vi "process camera timestamp.vi"(0 "Progress:":refnum<vi>, 1 "Use Harp converted .csv file\nto timestamp the file:":bool, 2 "abort":refnum<vi>, 3 "Register Address:":refnum<vi>, 4 "cam .csv":path, 5 "CameraBitPosition":refnum<vi>, 6 "don't ask":bool, 7 "harp .bin":path) -> (8 "error":string="Frames on Harp file: ")   [LabVIEW 2010]
panel:
  out "Frames Acquired":i32
  out "Numeric":i32
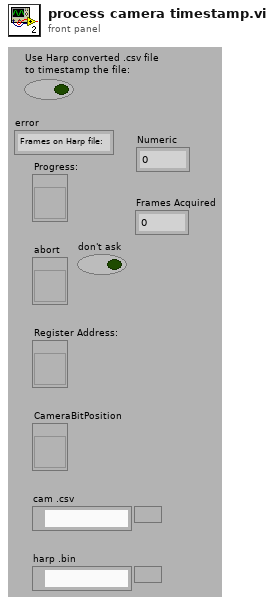
[diagram p1: front panel]
types:
  T1 = enum8{"Enabled", "Disabled", "Disabled and Grayed Out"}
  T2 = enum16{"open", "replace", "create", "open or create", "replace or create", "replace or create with confirmation"}
  T3 = enum16{"Left Button", "Center Button", "Right Button", "Window Close"}
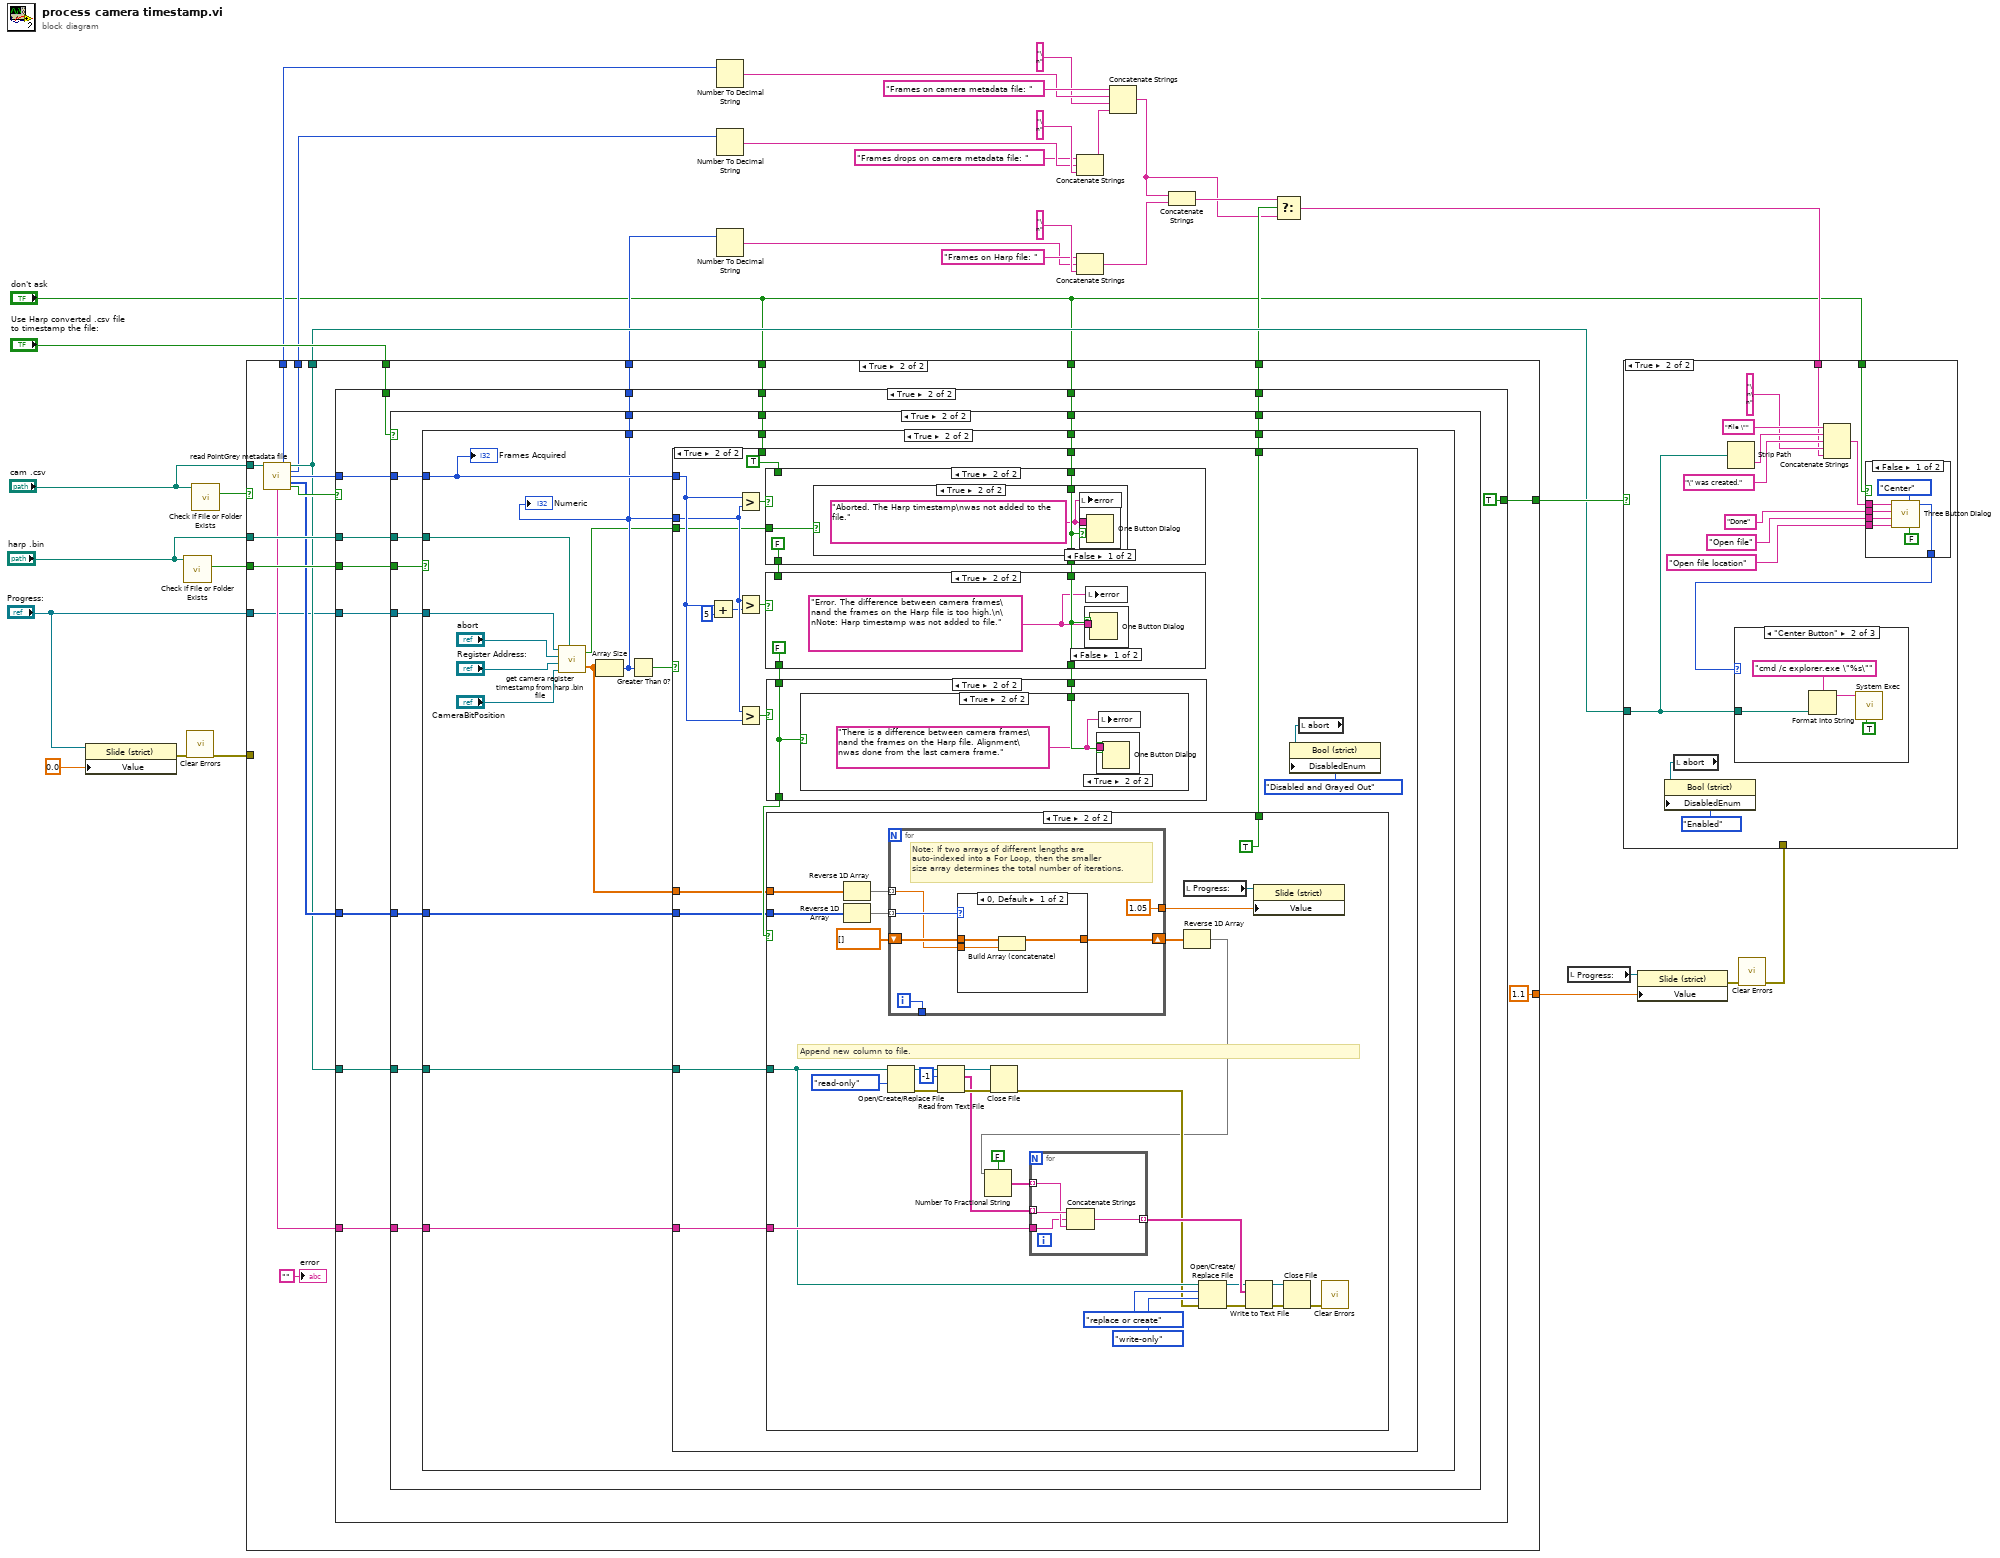
[diagram p0: block diagram]
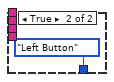
[diagram p3: hidden frame]
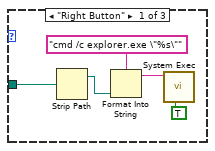
[diagram p4: hidden frame]
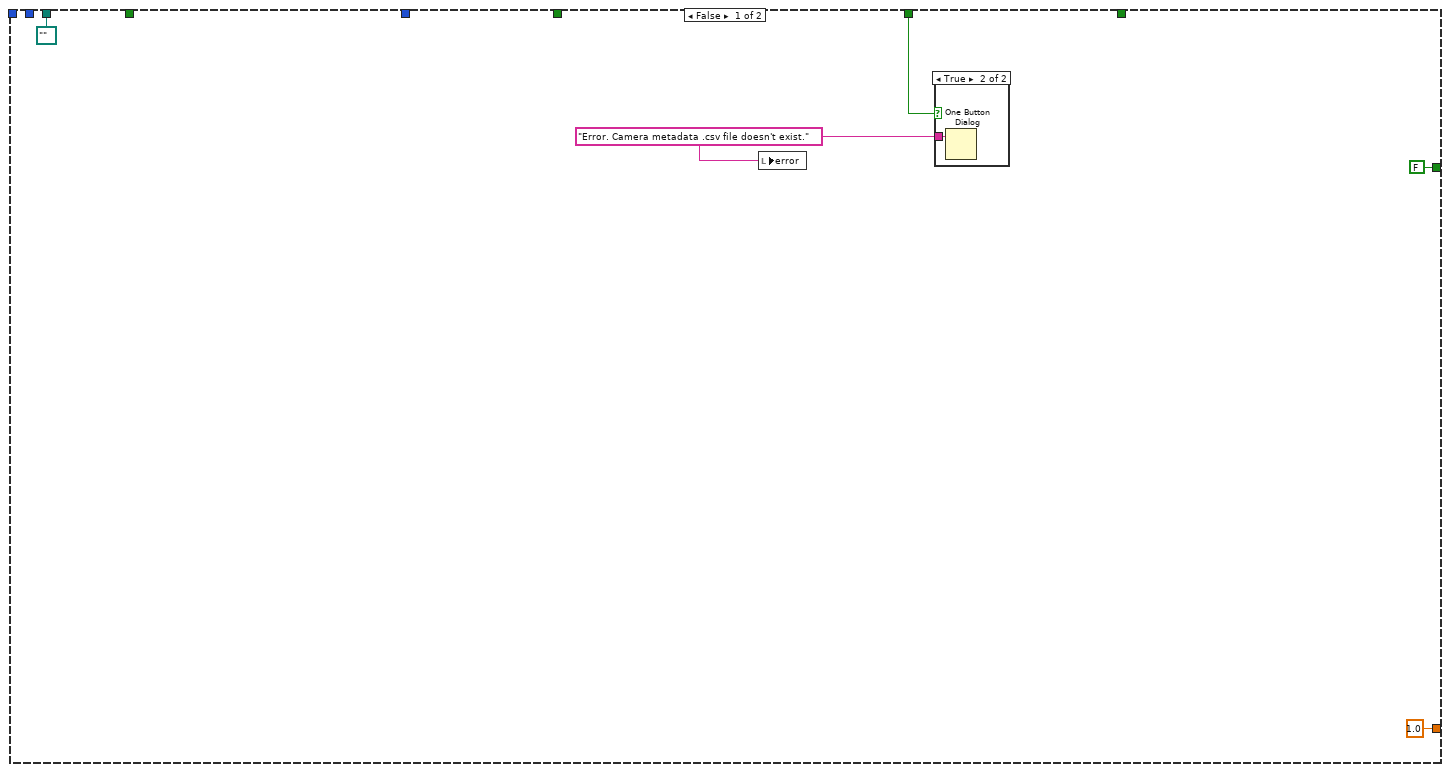
[diagram p6: hidden frame]
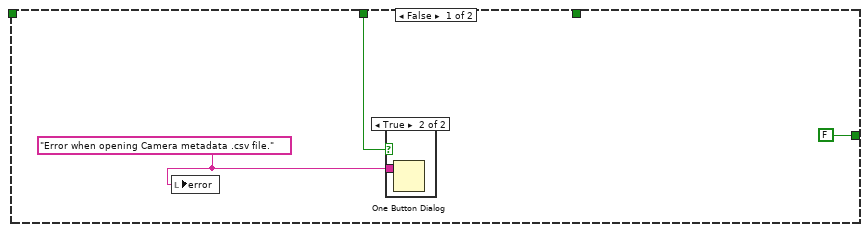
[diagram p8: hidden frame]
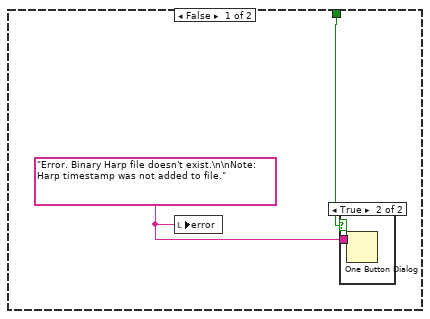
[diagram p11: hidden frame]
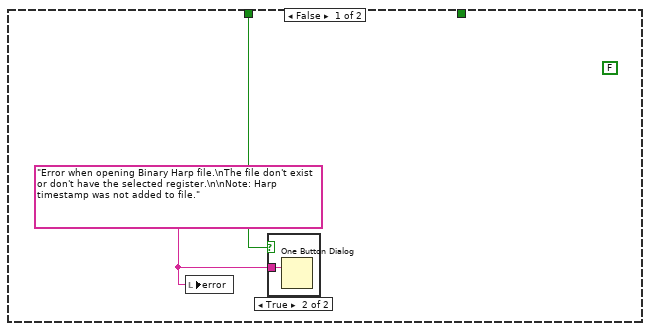
[diagram p13: hidden frame]
diagram:
  n1 = property class="Slide (strict)"(reference="Progress:", "Value"=0.0) -> (error out=w27:errorcluster)  [unwired: 1 in, 1 out]
  n2 = call <vilib>:"Check if File or Folder Exists.vi"("path"="harp .bin") -> ("file or folder exists?"=w30:bool)  [unwired: 8 in, 2 out]
  n3 = call <vilib>:"Clear Errors.vi"("error in (no error)"=w27) -> ("error out"=w26:errorcluster)  [unwired: 6 in]
  n4 = call <vilib>:"Check if File or Folder Exists.vi"("path"="cam .csv") -> ("file or folder exists?"=w33:bool)  [unwired: 8 in, 2 out]
  n5 = case shown="True" w33 {
    tunnel: "harp .bin" -> [_ w53]
    tunnel: "cam .csv" -> [_ w59]
    tunnel: "Use Harp converted .csv file\nto timestamp the file:" -> [_ w57]
    tunnel: [FALSE w56] -> w29
    tunnel: w30 -> [_ w55]
    tunnel: [path "" ("Created Csv File") w50] -> w28
    tunnel: w26 -> [_ _]
    tunnel: "Progress:" -> [_ w49]
    tunnel: [_ w48] -> w23
    tunnel: [_ w47] -> w16
    tunnel: [1.0 ("Value") 1.1 ("Value")] -> w10
    tunnel: [_ w45] -> w4
    tunnel: [_ w44] -> w2
    tunnel: "don't ask" -> [_ w43]
    tunnel: "don't ask" -> [w35 w42]
    frame False {
      w36 = "Error. Camera metadata .csv file doesn't exist." ("message")
      n6 = local write "error"(w36) -> ()
      n7 = case shown="True" w35 {
        tunnel: w36 -> [_ w40]
        frame False {
        }
        frame True {
          n8 = One Button Dialog(message=w40) -> ()  [unwired: 1 in, 1 out]
        }
      }
    }
    frame True {
      n9 = call "read PointGrey metadata file.vi"("PointGrey metadata file path"=w59) -> ("Frames On File"=w44:i32, "Created Csv File"=w50:path, "Frame Drops"=w45:i64, "Frames Acquired"=w54:i32, "FrameCounter (processed)"=w52:i64[], "Separation Character"=w51:string, "File Has Data"=w58:bool)  [unwired: 8 in]
      n10 = case shown="True" w58 {
        tunnel: w57 -> [_ w76]
        tunnel: [FALSE TRUE] -> w56
        tunnel: w55 -> [_ w75]
        tunnel: w54 -> [_ w66]
        tunnel: w53 -> [_ w74]
        tunnel: w52 -> [_ w73]
        tunnel: w50 -> [_ w72]
        tunnel: w51 -> [_ w71]
        tunnel: w49 -> [_ w69]
        tunnel: [_ w68] -> w48
        tunnel: [_ w67] -> w47
        tunnel: w43 -> [_ w65]
        tunnel: w42 -> [w60 w64]
        frame False {
          w61 = "Error when opening Camera metadata .csv file." ("message")
          n11 = local write "error"(w61) -> ()
          n12 = case shown="True" w60 {
            tunnel: w61 -> [_ w63]
            frame False {
            }
            frame True {
              n13 = One Button Dialog(message=w63) -> ()  [unwired: 1 in, 1 out]
            }
          }
        }
        frame True {
          n14 = case shown="True" w76 {
            tunnel: w75 -> [_ w87]
            tunnel: w66 -> [_ w86]
            tunnel: w74 -> [_ w85]
            tunnel: w73 -> [_ w84]
            tunnel: w72 -> [_ w83]
            tunnel: w71 -> [_ w82]
            tunnel: w69 -> [_ w81]
            tunnel: [_ w80] -> w68
            tunnel: [_ w79] -> w67
            tunnel: w65 -> [_ w78]
            tunnel: w64 -> [_ w77]
            frame False {
            }
            frame True {
              n15 = case shown="True" w87 {
                tunnel: w86 -> [_ w97]
                tunnel: w85 -> [_ w102]
                tunnel: w84 -> [_ w93]
                tunnel: w83 -> [_ w100]
                tunnel: w82 -> [_ w99]
                tunnel: w81 -> [_ w98]
                tunnel: [_ w96] -> w80
                tunnel: [_ w95] -> w79
                tunnel: w78 -> [_ w92]
                tunnel: w77 -> [w88 w91]
                frame False {
                  w89 = "Error. Binary Harp file doesn't exist.\n\nNote: Harp timestamp was not added to file." ("message")
                  n16 = local write "error"(w89) -> ()
                  n17 = case shown="True" w88 {
                    tunnel: w89 -> [_ w90]
                    frame False {
                    }
                    frame True {
                      n18 = One Button Dialog(message=w90) -> ()  [unwired: 1 in, 1 out]
                    }
                  }
                }
                frame True {
                  n19 = call "get camera register timestamp from harp .bin file.vi"("harp .bin"=w102, "reference 4"="CameraBitPosition", "reference 3"="Register Address:", "reference 2"="abort", "reference"=w98) -> ("Array"=w101:dbl[], "Abort"=w94:bool)  [unwired: 1 in]
                  n20 = Array Size(array=w101) -> (size(s)=w96:i32)
                  "Numeric" <- w96
                  n21 = Greater Than 0?(x=w96) -> (x > 0?=w103:bool)
                  n22 = case shown="True" w103 {
                    tunnel: w97 -> [_ w125]
                    tunnel: w96 -> [_ w118]
                    tunnel: w101 -> [_ w122]
                    tunnel: w93 -> [_ w121]
                    tunnel: w100 -> [_ w120]
                    tunnel: w99 -> [_ w119]
                    tunnel: [_ w116] -> w95
                    tunnel: w94 -> [_ w115]
                    tunnel: w92 -> [_ _]
                    tunnel: w91 -> [w108 w112]
                    frame False {
                      w107 = "Error when opening Binary Harp file.\nThe file don't exist or don't have the selected register.\n\nNote: Harp timestamp was not added to file." ("message")
                      (unwired) FALSE
                      n23 = local write "error"(w107) -> ()
                      n24 = case shown="True" w108 {
                        tunnel: w107 -> [_ w109]
                        frame False {
                        }
                        frame True {
                          n25 = One Button Dialog(message=w109) -> ()  [unwired: 1 in, 1 out]
                        }
                      }
                    }
                    frame True {
                      n26 = Add(x=w125, y=5) -> (x+y=w117:i32)
                      n27 = Greater?(x=w125, y=w118) -> (0:w131:bool)
                      n28 = Greater?(x=w118, y=w117) -> (0:w130:bool)
                      n29 = Greater?(x=w118, y=w125) -> (0:w124:bool)
                      n30 = case shown="True" w131 {
                        tunnel: [w189 FALSE] -> w128
                        tunnel: TRUE -> [w189 _]
                        tunnel: w115 -> [_ w192]
                        tunnel: w112 -> [w188 w191]
                        tunnel: [w188 w190] -> w111
                        frame False {
                        }
                        frame True {
                          n31 = case shown="True" w192 {
                            tunnel: w191 -> [w195 w198]
                            tunnel: [w195 w198] -> w190
                            frame False {
                              w194 = "Error. Camera has more frames than the Harp file.\n\nNote: Harp timestamp was not added to file." ("message")
                              n32 = case shown="False" w195 {
                                tunnel: w194 -> [w196 _]
                                frame False {
                                n33 = One Button Dialog(message=w196) -> ()  [unwired: 1 in, 1 out]
                                }
                                frame True {
                                }
                              }
                              n34 = local write "error"(w194) -> ()
                            }
                            frame True {
                              w197 = "Aborted. The Harp timestamp\nwas not added to the file." ("message")
                              n35 = local write "error"(w197) -> ()
                              n36 = case shown="False" w198 {
                                tunnel: w197 -> [w199 _]
                                frame False {
                                n37 = One Button Dialog(message=w199) -> ()  [unwired: 1 in, 1 out]
                                }
                                frame True {
                                }
                              }
                            }
                          }
                        }
                      }
                      n38 = case shown="True" w130 {
                        tunnel: [w183 FALSE] -> w126
                        tunnel: w128 -> [w183 _]
                        tunnel: w111 -> [w182 w185]
                        tunnel: [w182 w185] -> w110
                        frame False {
                        }
                        frame True {
                          w184 = "Error. The difference between camera frames\nand the frames on the Harp file is too high.\n\nNote: Harp timestamp was not added to file." ("message")
                          n39 = case shown="False" w185 {
                            tunnel: w184 -> [w187 _]
                            frame False {
                              n40 = One Button Dialog(message=w187) -> ()  [unwired: 1 in, 1 out]
                            }
                            frame True {
                            }
                          }
                          n41 = local write "error"(w184) -> ()
                        }
                      }
                      n42 = case shown="True" w124 {
                        tunnel: [w176 w178] -> w123
                        tunnel: w126 -> [w176 w178]
                        tunnel: w110 -> [_ w177]
                        frame False {
                        }
                        frame True {
                          n43 = case shown="True" w178 {
                            tunnel: w177 -> [_ w180]
                            frame False {
                            }
                            frame True {
                              w179 = "There is a difference between camera frames\nand the frames on the Harp file. Alignment\nwas done from the last camera frame." ("message")
                              n44 = case shown="True" w180 {
                                tunnel: w179 -> [_ w181]
                                frame False {
                                }
                                frame True {
                                n45 = One Button Dialog(message=w181) -> ()  [unwired: 1 in, 1 out]
                                }
                              }
                              n46 = local write "error"(w179) -> ()
                            }
                          }
                        }
                      }
                      n47 = case shown="True" w123 {
                        tunnel: w122 -> [_ w161]
                        tunnel: w121 -> [_ w157]
                        tunnel: w120 -> [_ w142]
                        tunnel: w119 -> [_ w148]
                        tunnel: [_ TRUE] -> w116
                        frame False {
                        }
                        frame True {
                          # "Append new column to file."
                          n48 = Reverse 1D Array(array=w161) -> (reversed array=w160:dbl[])
                          n49 = Reverse 1D Array(array=w157) -> (reversed array=w159:i64[])
                          n50 = Open/Create/Replace File(file path (use dialog)=w142, access (0:read/write)=enum16{"read/write", "read-only", "write-only"}."read-only") -> (refnum out=w155:refnum<file>, error out=w156:errorcluster)  [unwired: 4 in, 1 out]
                          n51 = for {
                            tunnel: w160 -> [w167] mode=indexing
                            tunnel: w159 -> [w171] mode=indexing
                            shift-right: [w170] -> w132
                            shift-left: dbl[] [] -> [w169]
                            tunnel: [1.05 ("Value")] -> w134
                            tunnel: [w166] -> _
                            i -> [w166]
                            # "Note: If two arrays of different lengths are\nauto-indexed into a For Loop, then the smaller\nsize array determines the total number of iterations."
                            n52 = case shown="0, Default" w171 {
                              tunnel: w167 -> [w174 _]
                              tunnel: [w173 w175] -> w170
                              tunnel: w169 -> [w172 w175]
                              frame 0, Default {
                                n53 = Build Array (concatenate)(w172, w174) -> (w173:dbl[])
                              }
                              frame -1 {
                              }
                            }
                          }
                          n54 = Read from Text File(file (use dialog)=w155, count=-1, error in=w156) -> (refnum out=w151:refnum<file>, text=w149:string[], error out=w152:errorcluster)  [unwired: 1 in, 1 out]
                          n55 = Close File(refnum=w151, error in=w152) -> (error out=w138:errorcluster)  [unwired: 1 out]
                          n56 = Reverse 1D Array(array=w132) -> (reversed array=w133:dbl[])
                          n57 = Number To Fractional String(use system decimal point (T)=FALSE, number=w133) -> (F-format string=w150:string[])  [unwired: 2 in]
                          n58 = for {
                            tunnel: w149 -> [w165] mode=indexing
                            tunnel: w150 -> [w164] mode=indexing
                            tunnel: [w163] -> w141 mode=indexing
                            tunnel: w148 -> [w162]
                            n59 = Concatenate Strings(w165, w162, w164) -> (w163:string)
                          }
                          n60 = local read "Progress:"() -> (w135:refnum<vi>)
                          n61 = Open/Create/Replace File(file path (use dialog)=w142, error in=w138, operation (0:open)=T2."replace or create", access (0:read/write)=enum16{"read/write", "read-only", "write-only"}."write-only") -> (refnum out=w140:refnum<file>, error out=w144:errorcluster)  [unwired: 2 in, 1 out]
                          n62 = Write to Text File(file (use dialog)=w140, text=w141, error in=w144) -> (refnum out=w139:refnum<file>, error out=w146:errorcluster)  [unwired: 1 in, 1 out]
                          n63 = property class="Slide (strict)"(reference=w135, "Value"=w134) -> ()  [unwired: 1 in, 2 out]
                          n64 = Close File(refnum=w139, error in=w146) -> (error out=w147:errorcluster)  [unwired: 1 out]
                          n65 = call <vilib>:"Clear Errors.vi"("error in (no error)"=w147) -> ()  [unwired: 6 in, 1 out]
                        }
                      }
                      n66 = local read "abort"() -> (w114:refnum<vi>)
                      n67 = property class="Bool (strict)"(reference=w114, "DisabledEnum"=T1."Disabled and Grayed Out" ("Disabled")) -> ()  [unwired: 1 in, 2 out]
                    }
                  }
                  "Frames Acquired" <- w97
                }
              }
            }
          }
        }
      }
      "error" <- ""
    }
  }
  n68 = Number To Decimal String(number=w2) -> (decimal integer string=w21:string)  [unwired: 1 in]
  n69 = Number To Decimal String(number=w4) -> (decimal integer string=w6:string)  [unwired: 1 in]
  n70 = Number To Decimal String(number=w23) -> (decimal integer string=w17:string)  [unwired: 1 in]
  n71 = Concatenate Strings("Frames drops on camera metadata file: " ("string"), w6, "\n" ("string")) -> (w3:string)
  n72 = Concatenate Strings("Frames on Harp file: " ("string"), w17, "\n" ("string")) -> (w14:string)
  n73 = Concatenate Strings("Frames on camera metadata file: " ("string"), w21, "\n" ("string"), w3) -> (w8:string)
  n74 = Concatenate Strings(w8, w14) -> (w15:string)
  n75 = Select(t=w15, s=w16, f=w8) -> (s? t:f=w13:string)
  n76 = local read "Progress:"() -> (w11:refnum<vi>)
  n77 = property class="Slide (strict)"(reference=w11, "Value"=w10) -> (error out=w12:errorcluster)  [unwired: 1 in, 1 out]
  n78 = call <vilib>:"Clear Errors.vi"("error in (no error)"=w12) -> ("error out"=w9:errorcluster)  [unwired: 6 in]
  n79 = case shown="True" w29 {
    tunnel: w28 -> [_ w213]
    tunnel: w13 -> [_ w203]
    tunnel: w9 -> [_ _]
    tunnel: "don't ask" -> [_ w200]
    frame False {
    }
    frame True {
      n80 = local read "abort"() -> (w201:refnum<vi>)
      n81 = property class="Bool (strict)"(reference=w201, "DisabledEnum"=T1."Enabled" ("Disabled")) -> ()  [unwired: 1 in, 2 out]
      n82 = Strip Path(path=w213) -> (name=w207:string)  [unwired: 1 out]
      n83 = Concatenate Strings("File \"" ("message"), w207, "\" was created." ("string"), "\n\n" ("string"), w203) -> (w205:string)
      n84 = case shown="False" w200 {
        tunnel: "Done" ("T button name (\"OK\")") -> [w220 _]
        tunnel: "Open file" ("F button name (\"Cancel\")") -> [w219 _]
        tunnel: "Open file location" ("F button name (\"Cancel\")") -> [w218 _]
        tunnel: [w216 T3."Left Button" ("Which Button?")] -> w209
        tunnel: w205 -> [w215 _]
        frame False {
          n85 = call <vilib>:"Three Button Dialog.vi"("Allow user to close window? (TRUE)"=FALSE, "Justify Message (Left)"=enum16{"Left", "Center", "Right"}."Center", "Right Button Text (\"Cancel\")"=w218, "Center Button Text (\"No\")"=w219, "Left Button Text (\"Yes\")"=w220, "message"=w215) -> ("Which Button?"=w216:T3)  [unwired: 5 in]
        }
        frame True {
        }
      }
      n86 = case shown="\"Center Button\"" w209 {
        tunnel: w213 -> [w223 w227 _]
        frame "Right Button" {
          n87 = Strip Path(path=w223) -> (stripped path=w222:path)  [unwired: 1 out]
          n88 = Format Into String(format string="cmd /c explorer.exe \"%s\"", w222) -> (resulting string=w226:string)  [unwired: 2 in, 1 out]
          n89 = call <vilib>:"System Exec.vi"("run minimized? (F)"=TRUE, "command line"=w226) -> ()  [unwired: 6 in, 4 out]
        }
        frame "Center Button" {
          n90 = Format Into String(format string="cmd /c explorer.exe \"%s\"", w227) -> (resulting string=w230:string)  [unwired: 2 in, 1 out]
          n91 = call <vilib>:"System Exec.vi"("run minimized? (F)"=TRUE, "command line"=w230) -> ()  [unwired: 6 in, 4 out]
        }
        frame "Left Button", Default {
        }
      }
    }
  }
